vi "Import Parameters Configuration to New Ballard ARINC 429 Custom Device.vi"(6 "Hardware Configuration File":path=path "Support/HW_Rx00_Tx24_Scheduled and Dynamic Labels.xml", 7 "Parameters Configuration File":path=path "Support/Parameters in Scheduled and Dynamic Labels.xml", 10 "Output System Definition File":path=path "Support/Imported Ballard ARINC 429.nivssdf", 11 "Base System Definition File":path=path "Support/Base.nivssdf") -> (3 "Ballard ARINC 429 System Definition":path)   [LabVIEW 2020, in "Ballard ARINC 429 Scripting Examples.lvlib"]
doc: "Overview: Demonstrates using the Ballard ARINC 429 scripting API to configure the custom device by importing a parameters configuration file. \n\nInstructions:\n1. Specify the Parameters Configuration File. This parameters configuration file must be consistent with the schema published on the GitHub repo (https://github.com/ni/niveristand-ballard-arinc429-custom-device/blob/main/Docs/Parameters%20XML%20File/ARINC429_Parameters_XML_Schema.xsd). For successful deployment, the parameters configuration file must also be consistent with the hardware configuration file.\n2. Specify the Hardware Configuration File. The hardware configuration file must be consistent with the schema installed by the Ballard hardware driver at C:\\Program Files (x86)\\Astronics Ballard Technology LabVIEW Driver\\Help\\index.html.\n3. (VeriStand) Optionally, you may open the Ballard ARINC 429 System Definition in VeriStand, configure the PXI Linux RT Target, and deploy the scripted system definition to perform avionics bus communications with Ballard ARINC 429 hardware."
uses:
  Ballard ARINC 429 Scripting Examples.lvlib
  NationalInstruments.VeriStand.SystemDefinitionAPI
  <vilib>/addons/VeriStand Custom Device Scripting APIs/Ballard/ARINC 429/Custom Device Support/Scripting/Ballard/Ballard ARINC 429 Scripting.lvlib
panel:
  # "Overview: Demonstrates using the Ballard ARINC 429 scripting API to configure the custom device by importing a parameters configuration file. \n\nInstructions:\n1. Specify the Parameters Configuration File. This parameters configuration file must be consistent with the schema published on the GitHub repo (https://github.com/ni/niveristand-ballard-arinc429-custom-device/blob/main/Docs/Parameters%20XML%20File/ARINC429_Parameters_XML_Schema.xsd). For successful deployment, the parameters configuration file must also be consistent with the hardware configuration file.\n2. Specify the Hardware Configuration File. The hardware configuration file must be consistent with the schema installed by the Ballard hardware driver at C:\\Program Files (x86)\\Astronics Ballard Technology LabVIEW Driver\\Help\\index.html.\n3. (VeriStand) Optionally, you may open the Ballard ARINC 429 System Definition in VeriStand, configure the PXI Linux RT Target, and deploy the scripted system definition to perform avionics bus communications with Ballard ARINC 429 hardware."
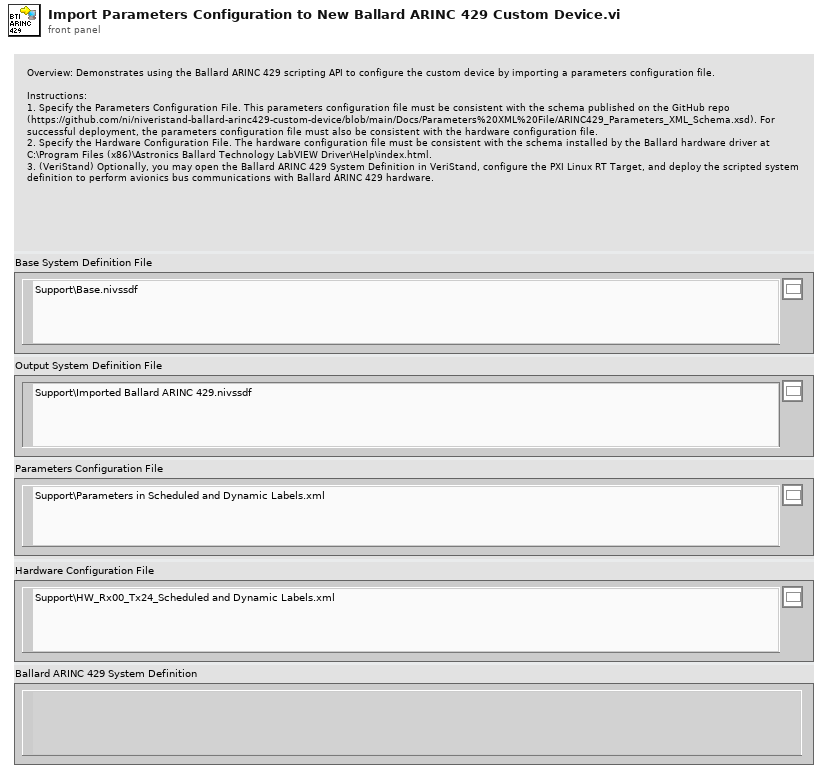
[diagram p1: front panel]
types:
  T1 = typedef "Custom Device API.lvlib/Custom Device Item Ref.ctl" = u64
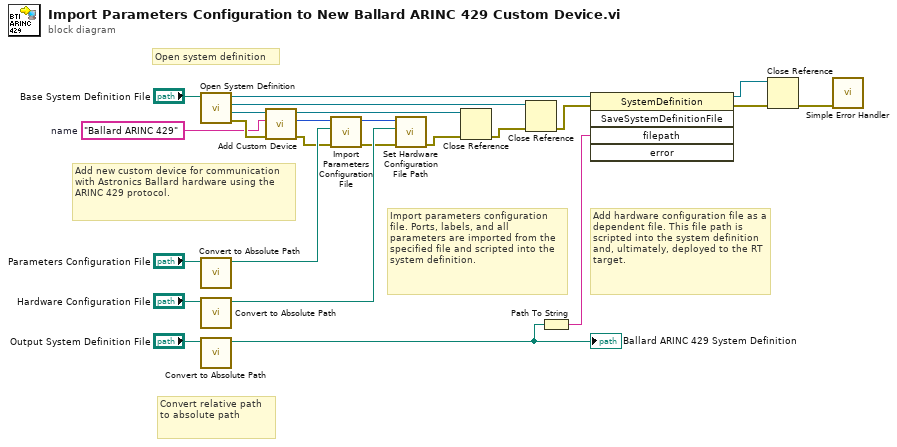
[diagram p0: block diagram]
diagram:
  w12 = "Ballard ARINC 429"  # name
  # "Add hardware configuration file as a dependent file. This file path is scripted into the system definition and, ultimately, deployed to the RT target."
  # "Import parameters configuration file. Ports, labels, and all parameters are imported from the specified file and scripted into the system definition."
  # "Add new custom device for communication with Astronics Ballard hardware using the ARINC 429 protocol."
  # "Convert relative path to absolute path"
  # "Open system definition"
  # "8."
  n1 = call "Open System Definition.vi"("System Definition File"="Base System Definition File") -> ("error out"=w13:errorcluster, "Target Refnum"=w14:refnum<k24>, "Root Refnum"=w16:refnum<k24>, "System Definition Refnum"=w17:refnum<k24>)  [unwired: 7 in]
  n2 = call "Convert to Absolute Path.vi"("System Definition File"="Parameters Configuration File") -> ("Absolute Path"=w10:path)  [unwired: 10 in]
  n3 = call "Convert to Absolute Path.vi"("System Definition File"="Hardware Configuration File") -> ("Absolute Path"=w8:path)  [unwired: 10 in]
  n4 = call "Convert to Absolute Path.vi"("System Definition File"="Output System Definition File") -> ("Absolute Path"=w1:path)  [unwired: 10 in]
  "Ballard ARINC 429 System Definition" <- w1
  n5 = call <vilib>:"Add Custom Device.vi"("error in"=w13, "name"=w12, "target in"=w14) -> ("error out"=w7:errorcluster, "Ballard ARINC 429 ref out"=w3:T1, "target out"=w2:refnum<k24>)  [unwired: 6 in]
  n6 = call <vilib>:"Import Parameters Configuration File.vi"("error in"=w7, "parameters configuration file path"=w10, "Ballard ARINC 429 ref"=w3) -> ("error out"=w5:errorcluster, "Ballard ARINC 429 ref out"=w6:T1)  [unwired: 7 in]
  n7 = call <vilib>:"Set Hardware Configuration File Path.vi"("error in"=w5, "path"=w8, "custom device ref"=w6) -> ("error out"=w4:errorcluster)  [unwired: 7 in, 1 out]
  n8 = Close Reference(reference=w2, error in (no error)=w4) -> (error out=w15:errorcluster)
  n9 = Close Reference(reference=w16, error in (no error)=w15) -> (error out=w20:errorcluster)
  n10 = Path To String(path=w1) -> (string=w23:string)
  n11 = invoke class="SystemDefinition" method="SaveSystemDefinitionFile"(reference=w17, error in=w20, "filepath"=w23) -> (reference out=w21:refnum<k24>, error out=w22:errorcluster)  [unwired: 2 in, 3 out]
  n12 = Close Reference(reference=w21, error in (no error)=w22) -> (error out=w19:errorcluster)
  n13 = call <vilib>:"Simple Error Handler.vi"("error in (no error)"=w19) -> ()  [unwired: 1 in, 8 out]
